vi "Main.vi"() -> ()   [LabVIEW 2017]
uses:
  Main.ctl
panel:
  out "Current count":i32
  in  "Reset Count":bool
  out "Status":T1=enum."Increment"
  in  "stop":bool
  in  "Input":cluster{"Target":i32}
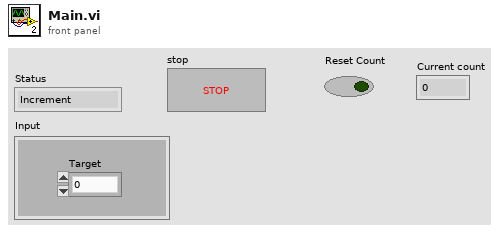
[diagram p1: front panel]
types:
  T1 = typedef "Main.ctl" = enum16{"Read Input", "Stop", "Increment", "Decrement", "Reset"}
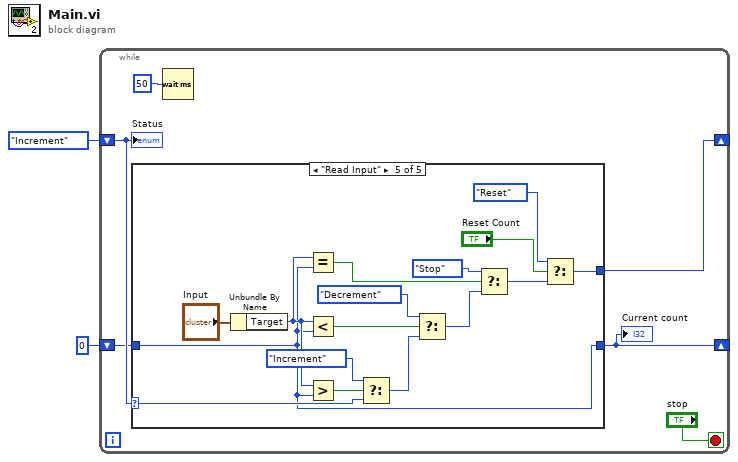
[diagram p0: block diagram]
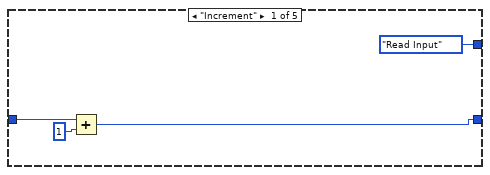
[diagram p2: hidden frame]
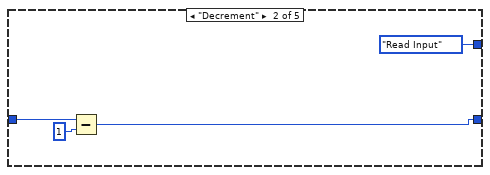
[diagram p3: hidden frame]
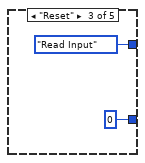
[diagram p4: hidden frame]
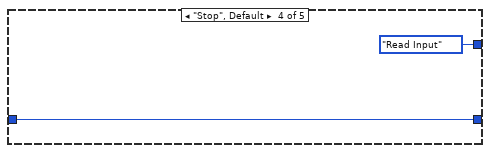
[diagram p5: hidden frame]
diagram:
  n1 = while {
    shift-right: [w5] -> _
    shift-left: 0 -> [w3]
    shift-right: [w4] -> _
    shift-left: Main."Increment" -> [w7]
    stop <- "stop" stop-if-true
    n2 = case shown="\"Read Input\"" w7 {
      selector: w7 -> [_ _ _ _ w22]
      tunnel: [w11 w15 0 ("Numeric") w20 w21] -> w5
      tunnel: [Main."Read Input" Main."Read Input" Main."Read Input" Main."Read Input" w23] -> w4
      tunnel: w3 -> [w10 w13 _ w20 w21]
      frame "Increment" {
        n3 = Add(x=w10, y=1) -> (x+y=w11:i32)
      }
      frame "Decrement" {
        n4 = Subtract(x=w13, y=1) -> (x-y=w15:i32)
      }
      frame "Reset" {
      }
      frame "Stop", Default {
      }
      frame "Read Input" {
        n5 = Unbundle By Name("Input") -> ("Target"=w34:i32)
        n6 = Equal?(x=w34, y=w21) -> (x = y?=w35:bool)
        n7 = Less?(x=w34, y=w21) -> (x < y?=w30:bool)
        n8 = Greater?(x=w34, y=w21) -> (0:w29:bool)
        n9 = Select(t=Main."Increment", s=w29, f=w22) -> (s? t:f=w31:T1)
        n10 = Select(t=Main."Decrement", s=w30, f=w31) -> (s? t:f=w33:T1)
        n11 = Select(t=Main."Stop", s=w35, f=w33) -> (s? t:f=w36:T1)
        n12 = Select(t=Main."Reset", s="Reset Count", f=w36) -> (s? t:f=w23:T1)
      }
    }
    "Current count" <- w5
    n13 = Wait (ms)(milliseconds to wait=u32 50) -> ()  [unwired: 1 out]
    "Status" <- w7
  }
